vi "update.vi"(3 "## (0)":u16, 5 "# (0)":u16, 6 "call chain index (1)":i32=1, 7 "vi ref (caller)":refnum<vi>, 8 "error in (no error)":errorcluster, 9 "?? (F)":bool, 10 "? (F)":bool, 11 "plan section":string) -> (0 "error out":errorcluster)   [LabVIEW 2024, in "controls manager.lvlib"]
uses:
  controls manager.lvlib
  selectors.ctl
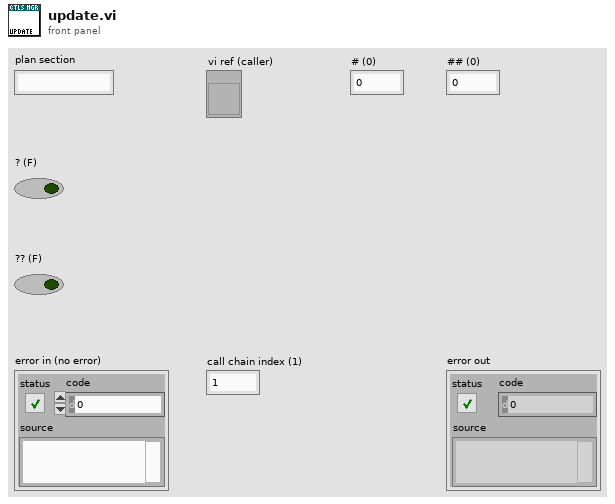
[diagram p1: front panel]
types:
  T1 = typedef "controls manager.lvlib/selectors.ctl" = cluster{"?":bool, "??":bool, "#":u16, "##":u16}
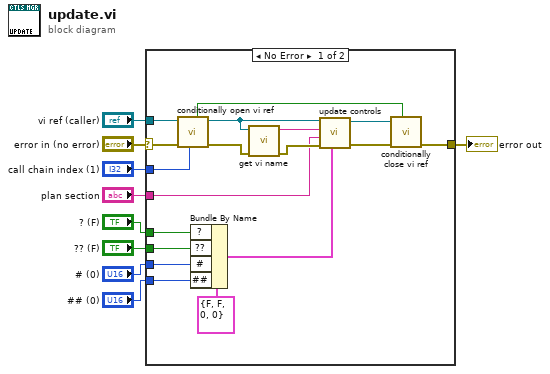
[diagram p0: block diagram]
diagram:
  n1 = case shown="No Error" "error in (no error)" {
    selector: "error in (no error)" -> [w25 w28]
    tunnel: "plan section" -> [w26 _]
    tunnel: [w22 w28] -> w8
    tunnel: "? (F)" -> [w18 _]
    tunnel: "?? (F)" -> [w17 _]
    tunnel: "# (0)" -> [w16 _]
    tunnel: "## (0)" -> [w15 _]
    tunnel: "vi ref (caller)" -> [w14 _]
    tunnel: "call chain index (1)" -> [w13 _]
    frame No Error {
      n2 = call "conditionally open vi ref.vi"("call chain index (1)"=w13, "error in (no error)"=w25, "vi ref in"=w14) -> ("error out"=w24:errorcluster, "vi ref out"=w12:refnum<vi>, "new ref?"=w21:bool)  [unwired: 6 in]
      n3 = Bundle By Name(cluster=T1 {"?"=FALSE, "??"=FALSE, "#"=0, "##"=0} ("selectors"), "?"=w18, "??"=w17, "#"=w16, "##"=w15) -> (w11:T1)
      n4 = call "get vi name.vi"("error in (no error)"=w24, "vi ref"=w12) -> ("error out"=w27:errorcluster, "vi name"=w20:string)  [unwired: 8 in]
      n5 = call "update controls.vi"("selectors"=w11, "error in (no error)"=w27, "plan section"=w26, "vi name"=w20, "vi ref in"=w12) -> ("error out"=w23:errorcluster, "vi ref out"=w10:refnum<vi>)  [unwired: 5 in]
      n6 = call "conditionally close vi ref.vi"("new ref?"=w21, "error in (no error)"=w23, "vi ref"=w10) -> ("error out"=w22:errorcluster)  [unwired: 8 in]
    }
    frame Error {
    }
  }
  "error out" <- w8
